vi "Read SubPanelReference.vi"(8 "error in (no error)":errorcluster, 11 "EmbeddedSMO in":refnum<class "EmbeddedSMO.lvclass">) -> (0 "error out":errorcluster, 2 "SubPanelReference":refnum<vi>, 3 "EmbeddedSMO out":refnum<class "EmbeddedSMO.lvclass">)   [LabVIEW 2016, in "EmbeddedSMO.lvclass"]
uses:
  EmbeddedSMO.lvclass
  EmbeddedSMO.lvclass/EmbeddedSMO.ctl
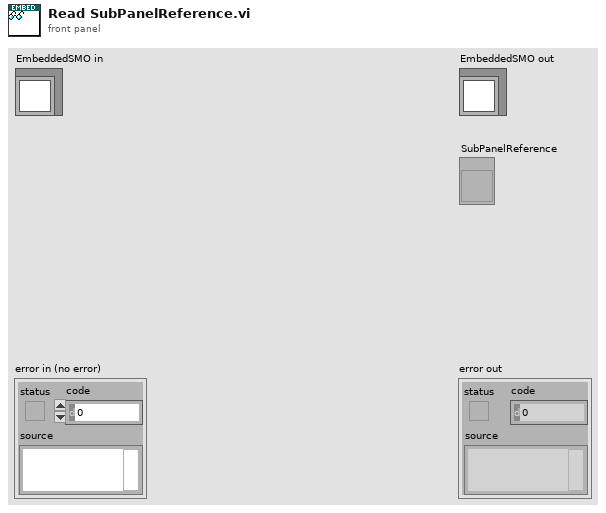
[diagram p1: front panel]
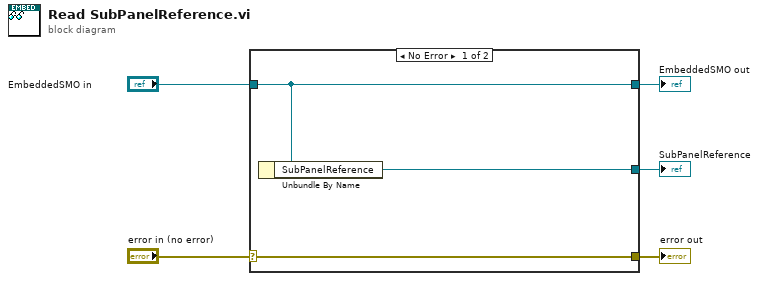
[diagram p0: block diagram]
diagram:
  n1 = case shown="No Error" "error in (no error)" {
    selector: "error in (no error)" -> [w8 w9]
    tunnel: [w8 w9] -> w4
    tunnel: [w7 w10] -> w2
    tunnel: "EmbeddedSMO in" -> [w7 w10]
    tunnel: [w6 _] -> w1
    frame No Error {
      n2 = Unbundle By Name(w7) -> ("SubPanelReference"=w6:refnum<vi>)
    }
    frame Error {
    }
  }
  "error out" <- w4
  "EmbeddedSMO out" <- w2
  "SubPanelReference" <- w1
